vi "Configure Active Trace.vi"(5 "Format":T1, 7 "S parameter":T2(ring), 8 "error in (no error)":errorcluster, 10 "Active Trace":u8=1, 11 "VNA-ZNB in":refnum<class "VNA-ZNB.lvclass">) -> (0 "error out":errorcluster, 3 "VNA-ZNB out":refnum<class "VNA-ZNB.lvclass">)   [LabVIEW 2020, in "VNA-ZNB.lvclass"]
doc: "Configures the active trace.\nIt creates the trace and sets the S paramert and mode."
uses:
  VNA-ZNB.lvclass
  C:/Sandbox/Git_Sandbox/WiSpry Test Framework source code (LV20)/WiSpry Test Framework/Instruments/Vector Network Analyzer/Vector Network Analyzer.lvclass
  C:/Sandbox/Git_Sandbox/WiSpry Test Framework source code (LV20)/WiSpry Test Framework/Instruments/Instrument.lvclass
  Controls/S parm format enum.ctl
  Vector Network Analyzer.lvclass/Vector Network Analyzer.ctl
  Instrument.lvclass/Instrument.ctl
  Vector Network Analyzer.lvclass
  Instrument.lvclass
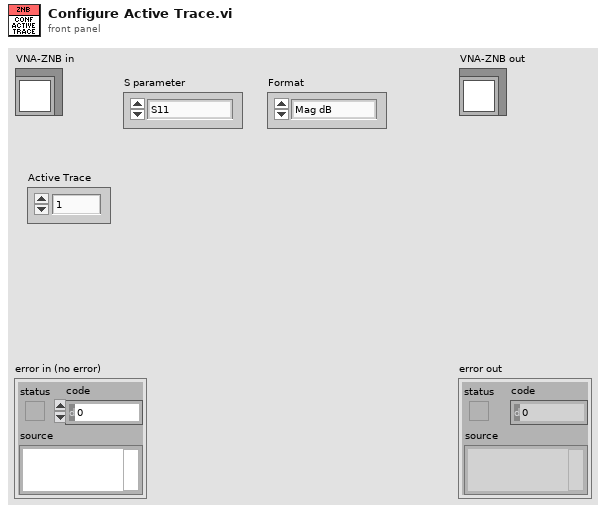
[diagram p1: front panel]
types:
  T1 = typedef "Vector Network Analyzer.lvclass/S parm format enum.ctl" = enum16{"Mag dB", "Mag", "Phase", "Smith", "Real", "Imag", "Group Delay", "SWR"}
  T2 = enum16{"S11", "S21", "S31", "S41", "S22", "S12", "S32", "S42", "S33", "S13", "S23", "S43", "S44", "S14", "S24", "S34"}
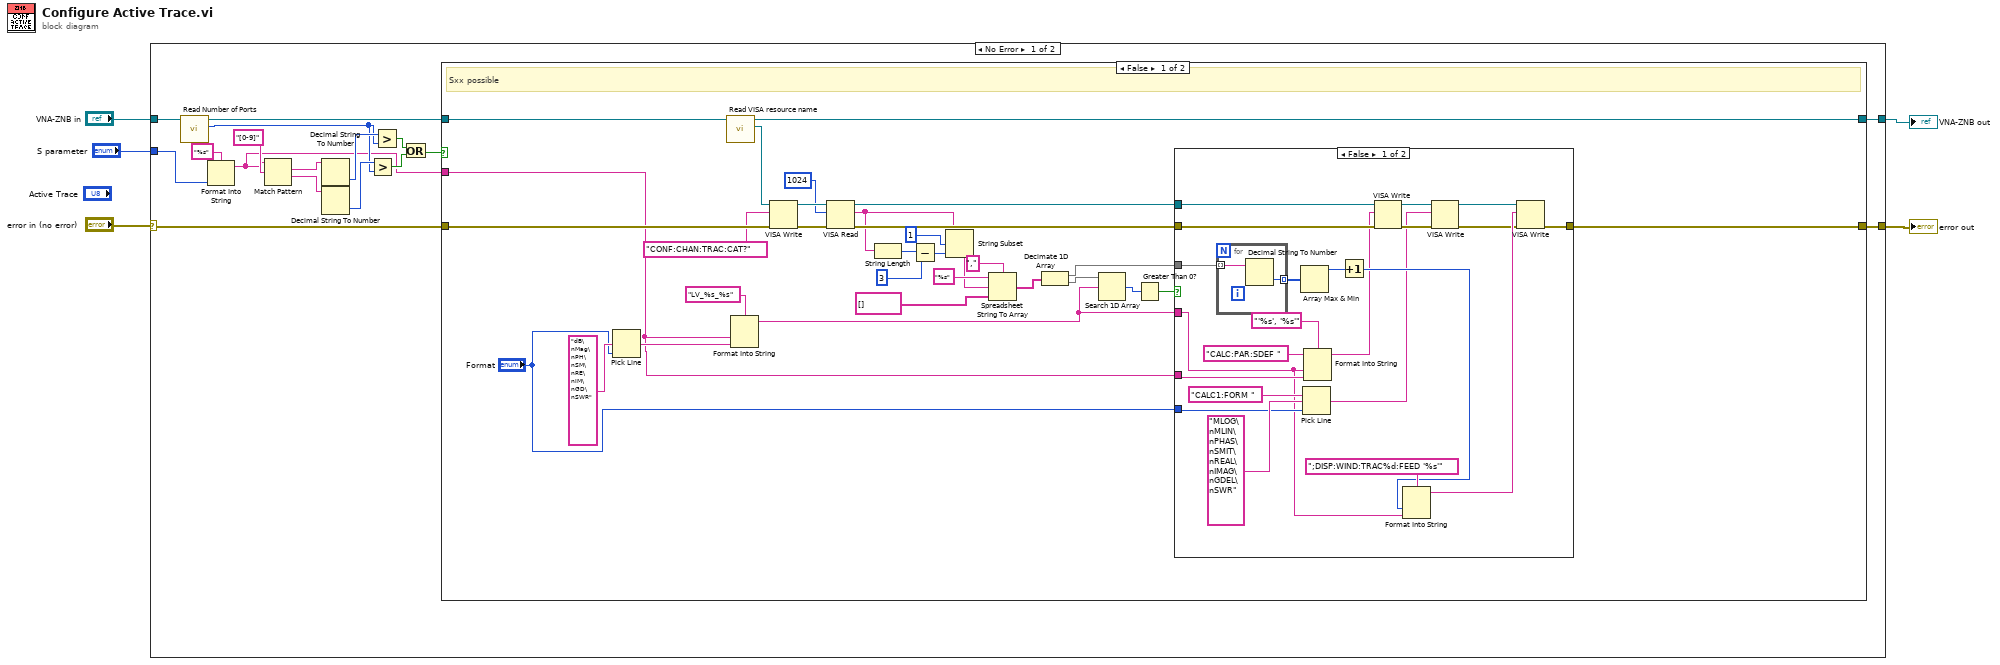
[diagram p0: block diagram]
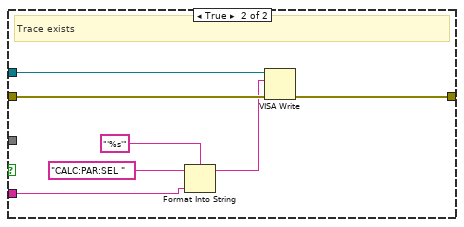
[diagram p2: hidden frame]
diagram:
  n1 = case shown="No Error" "error in (no error)" {
    selector: "error in (no error)" -> [w9 w88]
    tunnel: "VNA-ZNB in" -> [w22 w87]
    tunnel: "S parameter" -> [w20 _]
    tunnel: [w7 w88] -> w2
    tunnel: [w6 w87] -> w1
    frame No Error {
      n2 = call "Read Number of Ports.vi"("Vector Network Analyzer in"=w22) -> ("Number of Ports"=w14:i32, "Vector Network Analyzer out"=w10:refnum<class "VNA-ZNB.lvclass">)  [unwired: 9 in]
      n3 = Format Into String(format string="%s", w20) -> (resulting string=w8:string)  [unwired: 2 in, 1 out]
      n4 = Match Pattern(string=w8, regular expression="[0-9]") -> (match substring=w18:string, after substring=w17:string)  [unwired: 1 in, 2 out]
      n5 = Decimal String To Number(string=w18) -> (number=w16:i32)  [unwired: 2 in, 1 out]
      n6 = Decimal String To Number(string=w17) -> (number=w15:i32)  [unwired: 2 in, 1 out]
      n7 = Greater?(x=w15, y=w14) -> (0:w12:bool)
      n8 = Greater?(x=w16, y=w14) -> (0:w13:bool)
      n9 = Or(x=w13, y=w12) -> (x .or. y?=w11:bool)
      n10 = case shown="False" w11 {
        tunnel: w10 -> [w52 w86]
        tunnel: w9 -> [w51 w85]
        tunnel: w8 -> [w29 _]
        tunnel: [w31 w85] -> w7
        tunnel: [w49 w86] -> w6
        frame False {
          # "Sxx possible"
          n11 = Pick Line(multi-line string="dB\nMag\nPH\nSM\nRE\nIM\nGD\nSWR", line index="Format") -> (output string=w47:string)  [unwired: 1 in]
          n12 = call "Read VISA resource name.vi"("Instrument in"=w52) -> ("VISA resource name"=w50:refnum<visa-resource-name>, "Instrument out"=w49:refnum<class "VNA-ZNB.lvclass">)  [unwired: 9 in]
          n13 = Format Into String(format string="LV_%s_%s" ("initial string"), w29, w47) -> (resulting string=w34:string)  [unwired: 2 in, 1 out]
          n14 = VISA Write(VISA resource name=w50, write buffer="CONF:CHAN:TRAC:CAT?", error in (no error)=w51) -> (VISA resource name out=w44:refnum<visa-resource-name>, error out=w45:errorcluster)  [unwired: 1 out]
          n15 = VISA Read(VISA resource name=w44, byte count=u32 1024, error in (no error)=w45) -> (VISA resource name out=w33:refnum<visa-resource-name>, read buffer=w26:string, error out=w32:errorcluster)  [unwired: 1 out]
          n16 = String Length(string=w26) -> (length=w25:i32)
          n17 = Subtract(x=w25, y=3) -> (x-y=w23:i32)
          n18 = String Subset(string=w26, offset (0)=1, length (rest)=w23) -> (substring=w28:string)
          n19 = Spreadsheet String To Array(delimiter (Tab)=",", format string="%s", spreadsheet string=w28, array type (2D Dbl)=string[] []) -> (array=w39:string[])
          n20 = Decimate 1D Array(w39) -> (w36:string[], w38:string[])
          n21 = Search 1D Array(1D array=w38, element=w34) -> (index of element=w35:i32)  [unwired: 1 in]
          n22 = Greater Than 0?(x=w35) -> (x > 0?=w37:bool)
          n23 = case shown="False" w37 {
            tunnel: w36 -> [w72 _]
            tunnel: w34 -> [w64 w82]
            tunnel: w33 -> [w65 w80]
            tunnel: w32 -> [w62 w81]
            tunnel: [w57 w78] -> w31
            tunnel: "Format" -> [w73 _]
            tunnel: w29 -> [w67 _]
            frame False {
              n24 = for {
                tunnel: w72 -> [w77] mode=indexing
                tunnel: [w76] -> w71 mode=indexing
                n25 = Decimal String To Number(string=w77) -> (number=w76:i32)  [unwired: 2 in, 1 out]
              }
              n26 = Array Max & Min(array=w71) -> (max value=w70:i32)  [unwired: 3 out]
              n27 = Pick Line(string ("")="CALC1:FORM ", multi-line string="MLOG\nMLIN\nPHAS\nSMIT\nREAL\nIMAG\nGDEL\nSWR", line index=w73) -> (output string=w58:string)
              n28 = Format Into String(format string="'%s', '%s'", initial string="CALC:PAR:SDEF ", w64, w67) -> (resulting string=w61:string)  [unwired: 1 in, 1 out]
              n29 = Increment(x=w70) -> (x+1=w63:i32)
              n30 = VISA Write(VISA resource name=w65, write buffer=w61, error in (no error)=w62) -> (VISA resource name out=w60:refnum<visa-resource-name>, error out=w59:errorcluster)  [unwired: 1 out]
              n31 = Format Into String(format string=";DISP:WIND:TRAC%d:FEED '%s'" ("write buffer"), w63, w64) -> (resulting string=w55:string)  [unwired: 2 in, 1 out]
              n32 = VISA Write(VISA resource name=w60, write buffer=w58, error in (no error)=w59) -> (VISA resource name out=w56:refnum<visa-resource-name>, error out=w54:errorcluster)  [unwired: 1 out]
              n33 = VISA Write(VISA resource name=w56, write buffer=w55, error in (no error)=w54) -> (error out=w57:errorcluster)  [unwired: 2 out]
            }
            frame True {
              # "Trace exists"
              n34 = Format Into String(format string="'%s'", initial string="CALC:PAR:SEL ", w82) -> (resulting string=w79:string)  [unwired: 1 in, 1 out]
              n35 = VISA Write(VISA resource name=w80, write buffer=w79, error in (no error)=w81) -> (error out=w78:errorcluster)  [unwired: 2 out]
            }
          }
        }
        frame True {
          # "Add error handler"
          # "Sxx higher than ports"
        }
      }
    }
    frame Error {
    }
  }
  "error out" <- w2
  "VNA-ZNB out" <- w1
